vi "processNodes.vi"(8 "error in (no error)":errorcluster, 9 "Calling VI Reference i":refnum<vi>, 10 "Nodes[]":refnum<vi>[](array[refnum]), 11 "Node in":refnum<class "Node.lvclass">) -> (0 "error out":errorcluster, 3 "Node out":refnum<class "Node.lvclass">)   [LabVIEW 2016, in "Node.lvclass"]
uses:
  Node.lvclass
  Node.lvclass/Node.ctl
  Search/Search.lvclass/Search.ctl
  INodeFactory/INodeFactory.lvclass
  Project/Project.lvclass
  Search/Search.lvclass
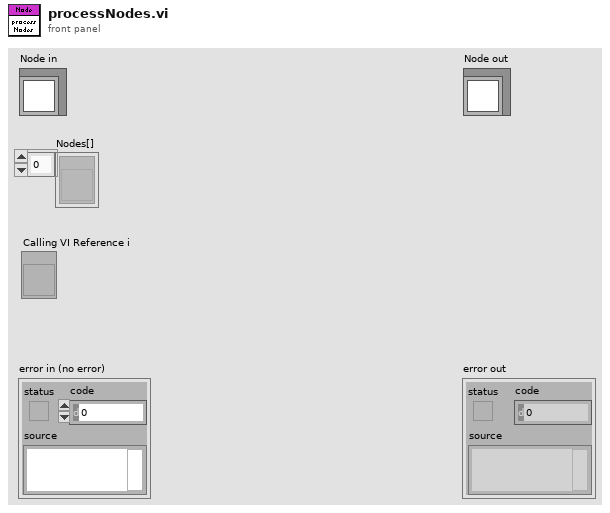
[diagram p1: front panel]
types:
  T1 = typedef "NodeSelection.ctl" = enum16{"Default", "CaseStructure", "EventStructure", "FlatSequence", "ForLoop", "WhileLoop"}
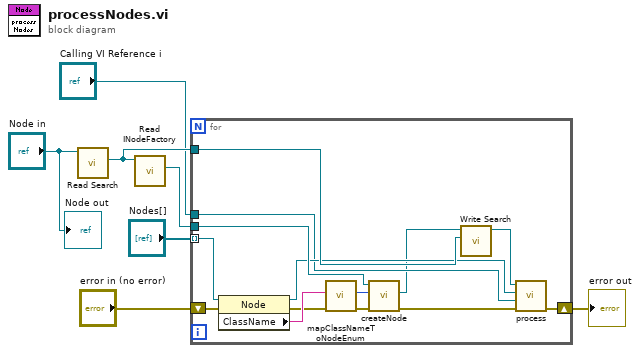
[diagram p0: block diagram]
diagram:
  n1 = call "Read Search.vi"("Node in"="Node in") -> ("Search"=w4:refnum<class "Search.lvclass">)  [unwired: 9 in, 1 out]
  n2 = call "Read INodeFactory.vi"("Search in"=w4) -> ("INodeFactory.lvclass"=w7:refnum<class "INodeFactory.lvclass">)  [unwired: 9 in, 1 out]
  n3 = for {
    tunnel: "Nodes[]" -> [w21] mode=indexing
    tunnel: w4 -> [w18]
    tunnel: w7 -> [w16]
    shift-right: [w11] -> w2
    shift-left: "error in (no error)" -> [w15]
    tunnel: "Calling VI Reference i" -> [w9]
    n4 = property class="Node"(reference=w21, error in=w15) -> (reference out=w10:refnum<vi>, error out=w14:errorcluster, "ClassName"=w20:string)
    n5 = call "mapClassNameToNodeEnum.vi"("error in (no error)"=w14, "Class Name"=w20) -> ("error out"=w13:errorcluster, "NodeSelection"=w19:T1)  [unwired: 7 in, 1 out]
    n6 = call-dynamic "createNode.vi"("error in (no error)"=w13, "NodeSelection"=w19, "INodeFactory in"=w16) -> ("error out"=w12:errorcluster, "Node"=w8:refnum<class "Node.lvclass">)  [unwired: 6 in, 1 out]
    n7 = call "Write Search.vi"("Search"=w18, "Node in"=w8) -> ("Node out"=w17:refnum<class "Node.lvclass">)  [unwired: 9 in]
    n8 = call-dynamic "process.vi"("error in (no error)"=w12, "Calling VI Reference i"=w9, "Node Refnum"=w10, "Node in"=w17) -> ("error out"=w11:errorcluster)  [unwired: 6 in, 1 out]
  }
  "error out" <- w2
  "Node out" <- "Node in"
